vi "DP_WebView_Create.vi"(0 "reference in":refnum<class "DP_WebView.lvclass">, 1 "Webview container":refnum<k24>(container), 2 "User Data Folder":path, 5 "Error In":errorcluster, 6 "Show Dialog if Run-Tim Engine is missing(True)":bool=TRUE) -> (12 "BrowserProcessId":u32, 13 "User Data Folder":path, 14 "reference out":refnum<class "DP_WebView.lvclass">, 15 "Status":i32(ring)=5 items=["Created", "WaitingForActivation", "WaitingToRun", "Running", "WaitingForChildrenToComplete", "RanToCompletion", "Canceled", "Faulted"], 16 "Status Message":string, 17 "Initialise Loops":i32=1, 18 "Reinstall Runtime":bool, 19 "Error Out":errorcluster)   [LabVIEW 2020, in "DP_WebView.lvclass"]
uses:
  DP_WebView.lvclass
  C:/Projects/DependencyViewer/DependencyViewer/DP_WebView_class/data/Microsoft.Web.WebView2.Wpf.dll
  data/Microsoft.Web.WebView2.Wpf.dll
  ctrls/ErrorCode.ctl
  C:/Projects/DependencyViewer/DependencyViewer/DP_WebView_class/data/Microsoft.Web.WebView2.Core.dll
  data/Microsoft.Web.WebView2.Core.dll
  C:/Projects/DependencyViewer/DependencyViewer/DP_WebView_class/data/Microsoft.Web.WebView2.WinForms.dll
  data/Microsoft.Web.WebView2.WinForms.dll
  data/WebView2Loader_32bit.dll
  data/WebView2Loader_64bit.dll
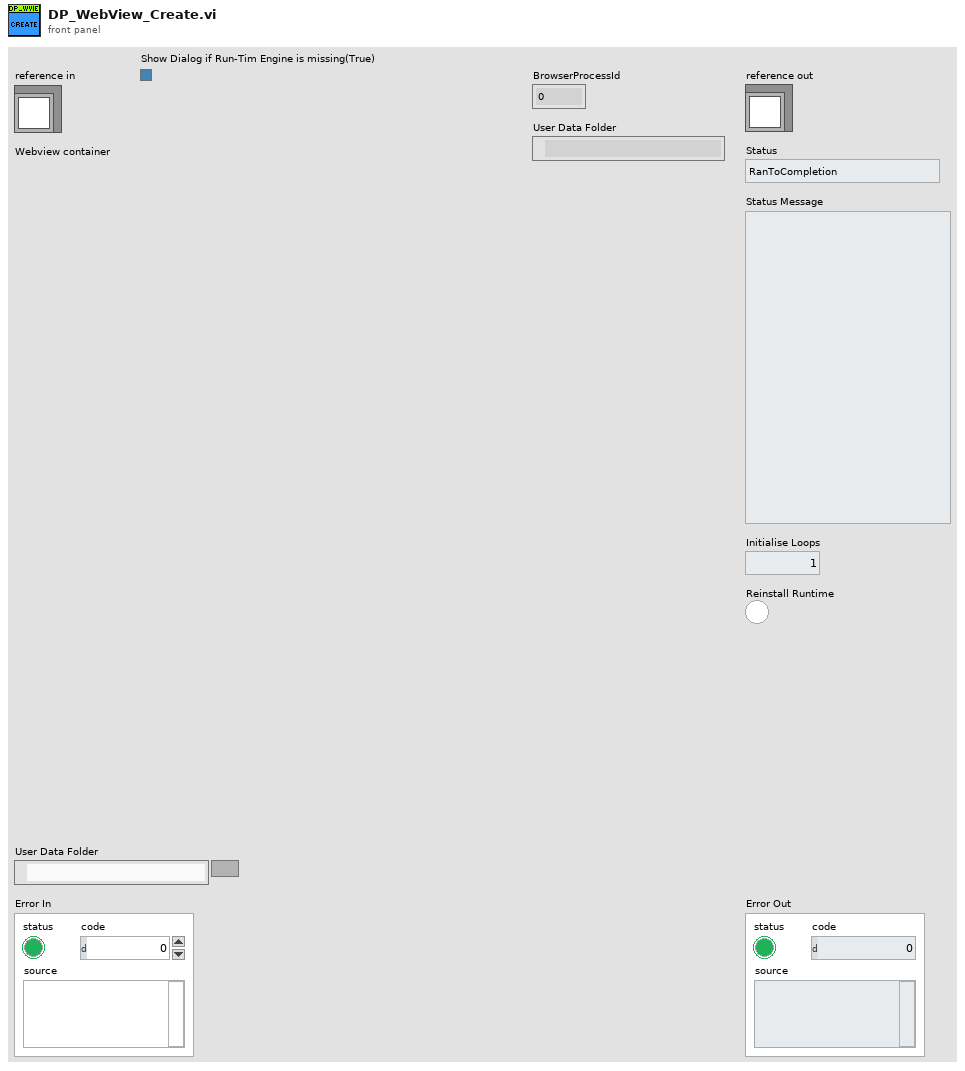
[diagram p1: front panel]
types:
  T1 = typedef "DP_WebView.lvclass/ErrorCode.ctl" = enum16{"Runtime engine is not installed or incompatible", "User Data Folder cannot be set", "Others", "JavaScript call failed", "PDF Printing Issue"}
  T2 = typedef "LcWebView.lvclass/ObjectAttributes.ctl" = cluster{"WebView Container":refnum<k24>, "CoreWebViewRef":refnum<k24>, "Status":i32, "Status Message":string, "User Data Folder":path, "BrowserProcessId":u32}
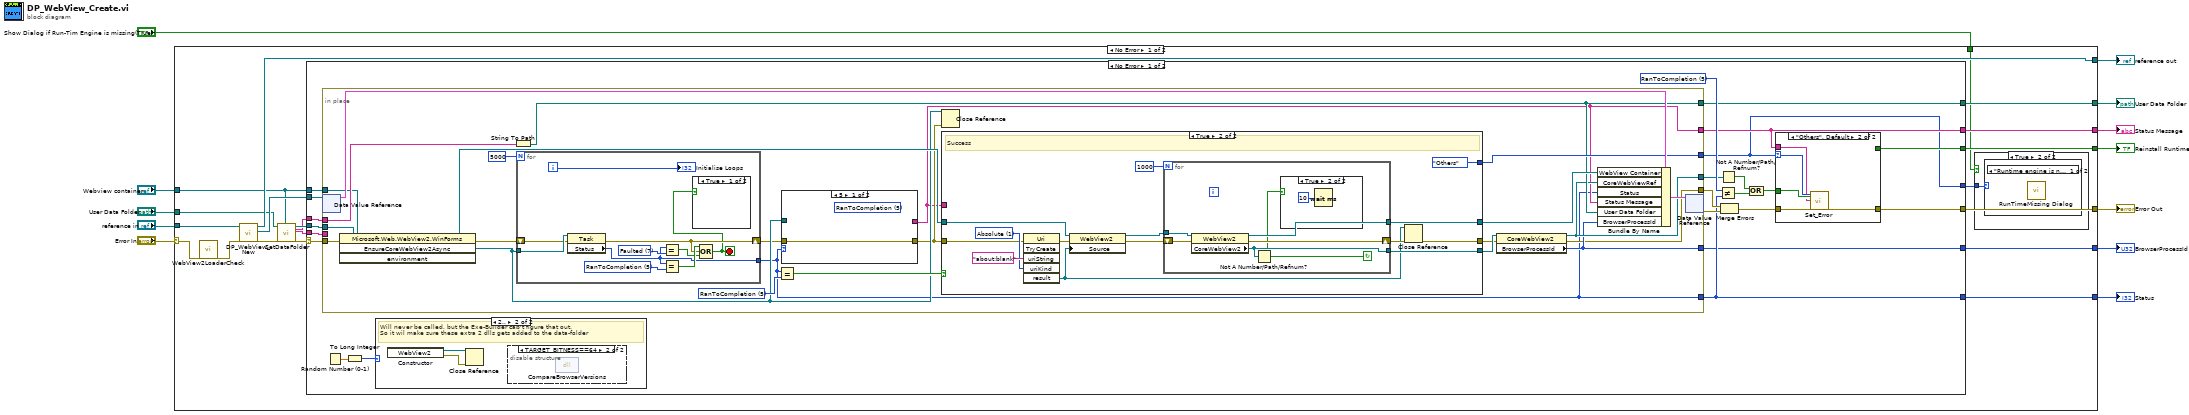
[diagram p0: block diagram]
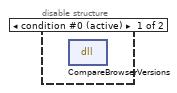
[diagram p5: hidden frame]
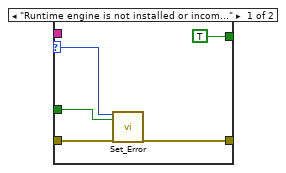
[diagram p6: hidden frame]
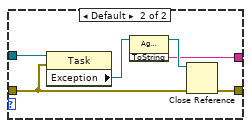
[diagram p7: hidden frame]
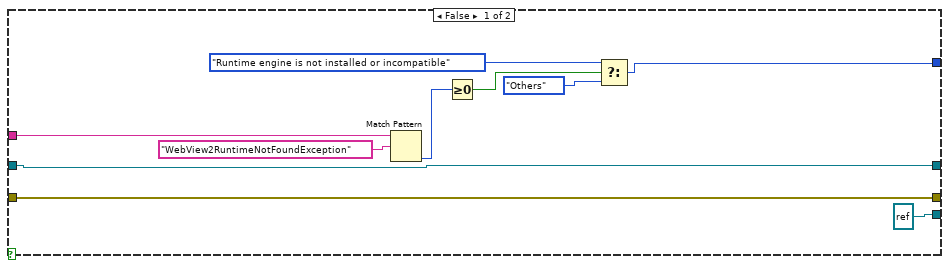
[diagram p8: hidden frame]
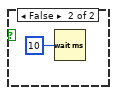
[diagram p10: hidden frame]
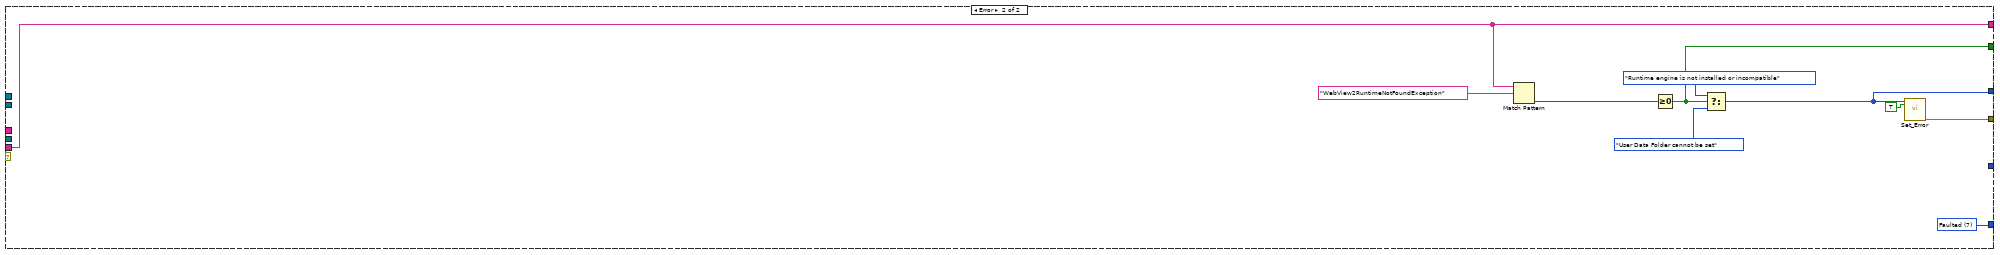
[diagram p11: hidden frame]
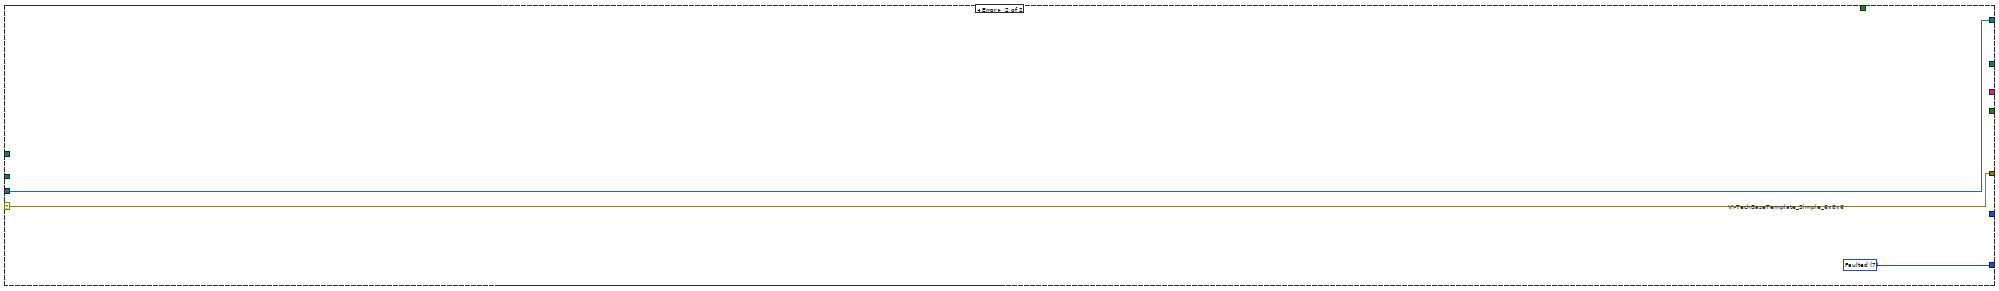
[diagram p12: hidden frame]
diagram:
  n1 = case shown="No Error" "Error In" {
    selector: "Error In" -> [w26 w154]
    tunnel: [w17 w154] -> w11
    tunnel: "reference in" -> [w32 w153]
    tunnel: [w31 w153] -> w9
    tunnel: [w29 w152] -> w8
    tunnel: [w28 _] -> w7
    tunnel: "Webview container" -> [w14 _]
    tunnel: [w27 _] -> w5
    tunnel: "User Data Folder" -> [w25 _]
    tunnel: [w19 _] -> w3
    tunnel: [w18 _] -> w2
    tunnel: "Show Dialog if Run-Tim Engine is missing(True)" -> [w15 _]
    frame No Error {
      n2 = call "WebView2LoaderCheck.vi"("Error In"=w26) -> ("Error Out"=w13:errorcluster)  [unwired: 18 in]
      n3 = call "DP_WebView_New.vi"("reference in"=w32, "error in (no error)"=w13) -> ("reference out"=w31:refnum<class "DP_WebView.lvclass">, "DVRRefOut"=w30:refnum<data-value>, "error out"=w22:errorcluster)  [unwired: 14 in, 1 out]
      n4 = call "SetDataFolder.vi"("User Data Folder"=w25, "error in (no error)"=w22, "Webview container"=w14) -> ("Environment"=w24:refnum<k24>, "UserDataFolder"=w20:string, "Error Message"=w21:string, "error out"=w23:errorcluster)  [unwired: 13 in]
      n5 = case shown="No Error" w23 {
        selector: w23 -> [w41 _]
        tunnel: w30 -> [w55 _]
        tunnel: [w53 w150] -> w29
        tunnel: w14 -> [w50 _]
        tunnel: [w45 w151] -> w17
        tunnel: [w44 w146] -> w28
        tunnel: [w43 w142] -> w27
        tunnel: w24 -> [w42 _]
        tunnel: w21 -> [w40 w146]
        tunnel: w20 -> [w39 _]
        tunnel: [w38 _] -> w19
        tunnel: [w37 _] -> w18
        tunnel: [w36 w143] -> w16
        frame No Error {
          w52 = 5 items=["Created", "WaitingForActivation", "WaitingToRun", "Running", "WaitingForChildrenToComplete", "RanToCompletion", "Canceled", "Faulted"] ("Status")
          n6 = in-place {
            in-place-border: w50 -> [w70]
            in-place-border: [w71] -> w53
            in-place-border: [w72] -> w44
            in-place-border: [w76] -> w54
            in-place-border: [w79] -> w49
            in-place-border: [w87] -> w36
            in-place-border: w42 -> [w81]
            in-place-border: w41 -> [w84]
            in-place-border: w40 -> [_]
            in-place-border: w39 -> [w83]
            in-place-border: [w82] -> w38
            in-place-border: [w77] -> w37
            w89 = 5 items=["Created", "WaitingForActivation", "WaitingToRun", "Running", "WaitingForChildrenToComplete", "RanToCompletion", "Canceled", "Faulted"] ("Status")
            n7 = in-place-dvr #1(w55) -> (w91:T2)  [unwired: 1 out]
            n8 = invoke class="Microsoft.Web.WebView2.WinForms" method="EnsureCoreWebView2Async"(reference=w70, error in=w84, "environment"=w81) -> (reference out=w85:refnum<k24>, error out=w69:errorcluster, "EnsureCoreWebView2Async"=w75:refnum<k24>)  [unwired: 1 in, 1 out]
            n9 = String To Path(string=w83) -> (path=w82:path)
            n10 = for {
              N: 5000 -> [_]
              tunnel: w75 -> [w140]
              shift-right: [w135] -> w74
              shift-left: w69 -> [w139]
              tunnel: [w133] -> w71
              i -> [w132]
              stop <- w131 stop-if-true
              w137 = 5 items=["Created", "WaitingForActivation", "WaitingToRun", "Running", "WaitingForChildrenToComplete", "RanToCompletion", "Canceled", "Faulted"] ("Status")
              w138 = 7 items=["Created", "WaitingForActivation", "WaitingToRun", "Running", "WaitingForChildrenToComplete", "RanToCompletion", "Canceled", "Faulted"] ("Status")
              n11 = property class="Task"(reference=w140, error in=w139) -> (error out=w135:errorcluster, "Status"=w133:i32)  [unwired: 1 out]
              n12 = Equal?(x=w133, y=w138) -> (x = y?=w134:bool)
              n13 = Equal?(x=w133, y=w137) -> (x = y?=w136:bool)
              n14 = Compound Arithmetic op=OR(w136, w135, w134) -> (w131:bool)
              n15 = case shown="True" w131 {
                frame True {
                }
                frame False {
                  n16 = Wait (ms)(milliseconds to wait=u32 10) -> ()  [unwired: 1 out]
                }
              }
              "Initialise Loops" <- w132
            }
            n17 = Equal?(x=w71, y=w89) -> (x = y?=w88:bool)
            n18 = case shown="5" w71 {
              tunnel: w75 -> [_ w99]
              tunnel: w74 -> [w93 w97]
              tunnel: [w93 w95] -> w73
              tunnel: [_ w94] -> w72
              frame 5 {
                (unwired) 5 items=["Created", "WaitingForActivation", "WaitingToRun", "Running", "WaitingForChildrenToComplete", "RanToCompletion", "Canceled", "Faulted"] ("Status")
              }
              frame Default {
                n19 = property class="Task"(reference=w99, error in=w97) -> ("Exception"=w98:refnum<k24>)  [unwired: 2 out]
                n20 = invoke class="AggregateException" method="ToString"(reference=w98) -> (reference out=w96:refnum<k24>, "ToString"=w94:string)  [unwired: 2 in, 1 out]
                n21 = Close Reference(reference=w96, error in (no error)=w97) -> (error out=w95:errorcluster)
              }
            }
            n22 = Close Reference(reference=w75, error in (no error)=w73) -> ()  [unwired: 1 out]
            n23 = case shown="True" w88 {
              tunnel: w73 -> [w107 w117]
              tunnel: [w109 w123] -> w86
              tunnel: [refnum<k24> refnum ("CoreWebView2") w122] -> w80
              tunnel: [w107 w111] -> w78
              tunnel: w85 -> [w109 w116]
              tunnel: w72 -> [w106 _]
              tunnel: [w100 ErrorCode."Others" ("f")] -> w87
              frame False {
                n24 = Match Pattern(string=w106, regular expression="WebView2RuntimeNotFoundException") -> (offset past match=w104:i32)  [unwired: 1 in, 3 out]
                n25 = Greater Or Equal To 0?(x=w104) -> (x >= 0?=w103:bool)
                n26 = Select(t=ErrorCode."Runtime engine is not installed or incompatible" ("CustomErrors"), s=w103, f=ErrorCode."Others") -> (s? t:f=w100:T1)
              }
              frame True {
                w118 = 1 items=["RelativeOrAbsolute", "Absolute", "Relative"] ("uriKind")
                # "Success"
                n27 = invoke class="Uri" method="TryCreate"(error in=w117, "uriString"="about:blank", "uriKind"=w118) -> (error out=w114:errorcluster, "result"=w110:refnum<k24>)  [unwired: 3 in, 4 out]
                n28 = property class="WebView2"(reference=w116, error in=w114, "Source"=w110) -> (reference out=w115:refnum<k24>, error out=w113:errorcluster)
                n29 = for {
                  N: 1000 -> [_]
                  tunnel: w115 -> [w129]
                  shift-right: [w127] -> w112
                  shift-left: w113 -> [w128]
                  tunnel: [w126] -> w122
                  tunnel: [w125] -> w123
                  stop <- w124 continue-if-true
                  n30 = property class="WebView2"(reference=w129, error in=w128) -> (reference out=w125:refnum<k24>, error out=w127:errorcluster, "CoreWebView2"=w126:refnum<k24>)
                  n31 = Not A Number/Path/Refnum?(number/path/refnum=w126) -> (NaN/Path/Refnum?=w124:bool)
                  n32 = case shown="True" w124 {
                    frame False {
                    }
                    frame True {
                      n33 = Wait (ms)(milliseconds to wait=u32 10) -> ()  [unwired: 1 out]
                    }
                  }
                }
                n34 = Close Reference(reference=w110, error in (no error)=w112) -> (error out=w111:errorcluster)
              }
            }
            n35 = property class="CoreWebView2"(reference=w80, error in=w78) -> (reference out=w79:refnum<k24>, error out=w76:errorcluster, "BrowserProcessId"=w77:u32)
            n36 = Bundle By Name(cluster=w91, "WebView Container"=w86, "CoreWebViewRef"=w79, "Status"=w71, "Status Message"=w72, "User Data Folder"=w82, "BrowserProcessId"=w77) -> (w92:T2)
            n37 = in-place-dvr #1(w92) -> (w56:errorcluster)  [unwired: 1 out]
          }
          n38 = Random Number (0-1)() -> (number: 0 to 1=w35:dbl)
          n39 = To Long Integer(number=w35) -> (32bit integer=w34:i32)
          n40 = case shown="2.." w34 {
            frame Default {
            }
            frame 2.. {
              # "Will never be called, but the Exe-Builder cab't figure that out.\nSo it wil make sure these extra 2 dlls gets added to the data-folder"
              n41 = constructor class="WebView2"() -> (reference out=w58:refnum<k24>, error out=w57:errorcluster)  [unwired: 3 in, 1 out]
              n42 = Close Reference(reference=w58, error in (no error)=w57) -> ()  [unwired: 1 out]
              n43 = disable-structure shown="TARGET_BITNESS==64" {
                frame condition #0 (active) {
                  n44 = dll-call lib="C:/Projects/DependencyViewer/DependencyViewer/DP_WebView_class/data/WebView2Loader_32bit.dll" fn="CompareBrowserVersions"() -> ()  [unwired: 4 in, 2 out]
                }
                frame condition #1 {
                  n45 = dll-call lib="C:/Projects/DependencyViewer/DependencyViewer/DP_WebView_class/data/WebView2Loader_64bit.dll" fn="CompareBrowserVersions"() -> ()  [unwired: 4 in, 2 out]
                }
              }
            }
          }
          n46 = Not Equal?(x=w52, y=w53) -> (x != y?=w51:bool)
          n47 = Not A Number/Path/Refnum?(number/path/refnum=w49) -> (NaN/Path/Refnum?=w48:bool)
          n48 = Merge Errors(w54, w56) -> (w47:errorcluster)
          n49 = Compound Arithmetic op=OR(w48, w51) -> (w46:bool)
          n50 = case shown="\"Others\", Default" w36 {
            selector: w36 -> [w61 w65]
            tunnel: w47 -> [w63 w68]
            tunnel: w46 -> [w60 w67]
            tunnel: [w62 w66] -> w45
            tunnel: w44 -> [_ w64]
            tunnel: [TRUE _] -> w43
            frame "Runtime engine is not installed or incompatible" {
              n51 = call "Set_Error.vi"("CustomErrors"=w61, "SetError(True)"=w60, "error in (no error)"=w63) -> ("error out"=w62:errorcluster)  [unwired: 16 in]
            }
            frame "Others", Default {
              n52 = call "Set_Error.vi"("CustomErrors"=w65, "SetError(True)"=w67, "Description"=w64, "error in (no error)"=w68) -> ("error out"=w66:errorcluster)  [unwired: 15 in]
            }
          }
        }
        frame Error {
          w150 = 7 items=["Created", "WaitingForActivation", "WaitingToRun", "Running", "WaitingForChildrenToComplete", "RanToCompletion", "Canceled", "Faulted"] ("Status")
          n53 = Match Pattern(string=w146, regular expression="WebView2RuntimeNotFoundException") -> (offset past match=w147:i32)  [unwired: 1 in, 3 out]
          n54 = Greater Or Equal To 0?(x=w147) -> (x >= 0?=w142:bool)
          n55 = Select(t=ErrorCode."Runtime engine is not installed or incompatible" ("CustomErrors"), s=w142, f=ErrorCode."User Data Folder cannot be set" ("CustomErrors")) -> (s? t:f=w143:T1)
          n56 = call "Set_Error.vi"("CustomErrors"=w143, "SetError(True)"=TRUE) -> ("error out"=w151:errorcluster)  [unwired: 17 in]
        }
      }
      n57 = case shown="True" w15 {
        tunnel: w16 -> [_ w33]
        frame False {
        }
        frame True {
          n58 = case shown="\"Runtime engine is not installed or incompatible\"" w33 {
            frame "Runtime engine is not installed or incompatible" {
              n59 = call "RunTimeMissing Dialog.vi"() -> ()  [unwired: 19 in, 1 out]
            }
            frame Default {
            }
          }
        }
      }
    }
    frame Error {
      w152 = 7 items=["Created", "WaitingForActivation", "WaitingToRun", "Running", "WaitingForChildrenToComplete", "RanToCompletion", "Canceled", "Faulted"] ("Status")
      # "VI-TechBaseTemplate_Simple_6x8x6"
    }
  }
  "Error Out" <- w11
  "reference out" <- w9
  "Status" <- w8
  "Status Message" <- w7
  "Reinstall Runtime" <- w5
  "User Data Folder" <- w3
  "BrowserProcessId" <- w2
